vi "Datasheet Generate (Dynamic).vi"(4 "Generator Settings":T3, 8 "error in (no error)":errorcluster, 10 "Templates":string[](array[string]), 11 "Items":T2[](array[typedef])) -> (0 "error out":errorcluster, 2 "Actual (sec)":i32, 3 "Datasheet Paths":T1[](array[typedef]))   [LabVIEW 2011]
uses:
  Datasheet Generator Settings.ctl
  www/cgi-bin/_cgi-lib/TDM_INDEX Record.ctl
  Datasheet Report Info.ctl
  Datasheet Inputs.ctl
  Datasheet Outputs.ctl
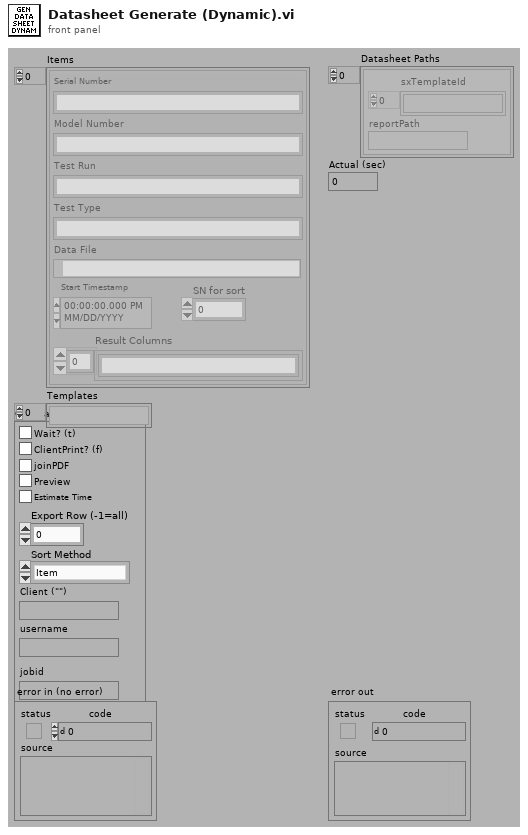
[diagram p1: front panel]
types:
  T1 = typedef "Datasheet Report Info.ctl" = cluster{"sxTemplateId":string[], "reportPath":path}
  T2 = typedef "TDM_INDEX Record.ctl" = cluster{"Model Number":string, "SN for sort":i32, "Test Type":string, "Test Run":string, "Serial Number":string, "Start Timestamp":timestamp, "Data File":path, "Result Columns":string[]}
  T3 = typedef "DATASHEET Generator Settings.ctl" = cluster{"Wait? (t)":bool, "ClientPrint? (f)":bool, "Client (\"\")":string, "joinPDF":bool, "Sort Method":enum16{"Item", "Template", "No Sort"}, "Export Row (-1=all)":i32, "Preview":bool, "Estimate Time":bool, "username":string, "jobid":string}
  T4 = typedef "Datasheet Outputs.ctl" = cluster{"Datasheet Paths":T5[], "Actual (Sec)":i32, "error out":errorcluster}
  T5 = typedef "DATASHEET Report Info.ctl" = cluster{"sxTemplateId":string[], "reportPath":path}
  T6 = typedef "DATASHEET INPUTS.ctl" = cluster{"Items":T2[], "Templates":string[], "Generator Settings":T3, "Response Queue Name":string}
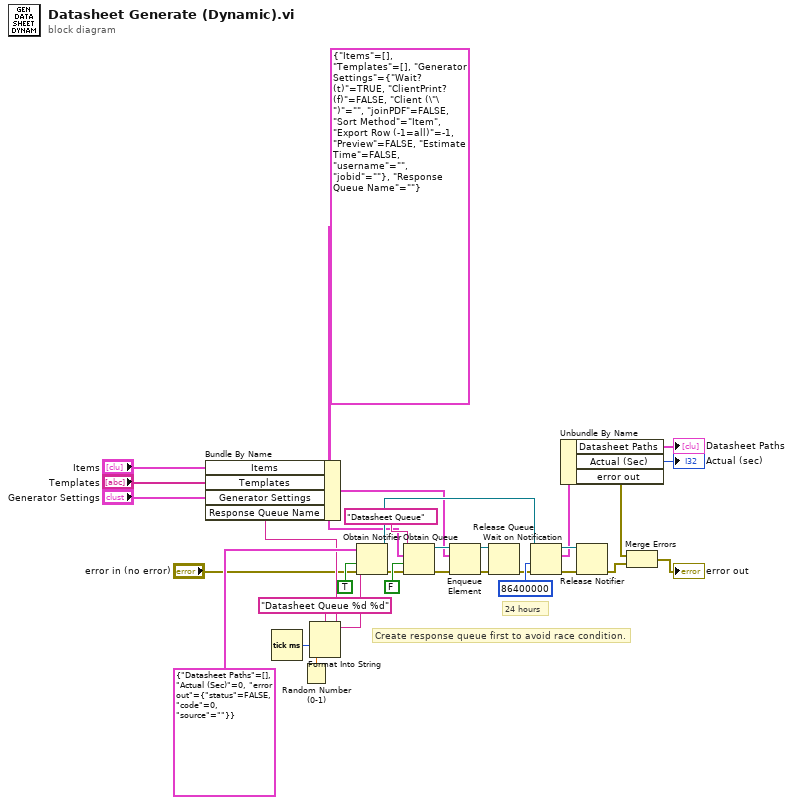
[diagram p0: block diagram]
diagram:
  w2 = T6 {"Items"=[], "Templates"=[], "Generator Settings"={"Wait? (t)"=TRUE, "ClientPrint? (f)"=FALSE, "Client (\"\")"="", "joinPDF"=FALSE, "Sort Method"=enum."Item", "Export Row (-1=all)"=-1, "Preview"=FALSE, "Estimate Time"=FALSE, "username"="", "jobid"=""}, "Response Queue Name"=""} ("INPUTS")
  # "Create response queue first to avoid race condition."
  # "24 hours"
  n1 = Tick Count (ms)() -> (millisecond timer value=w18:u32)
  n2 = Random Number (0-1)() -> (number: 0 to 1=w11:dbl)
  n3 = Format Into String(format string="Datasheet Queue %d %d" ("name (unnamed)"), w18, w11) -> (resulting string=w10:string)  [unwired: 2 in, 1 out]
  n4 = Bundle By Name(cluster=w2, "Items"="Items", "Templates"="Templates", "Generator Settings"="Generator Settings", "Response Queue Name"=w10) -> (w3:T6)
  n5 = Obtain Notifier(name (unnamed)=w10, notification data type=T4 {"Datasheet Paths"=[], "Actual (Sec)"=0, "error out"={"status"=FALSE, "code"=0, "source"=""}} ("OUTPUTS"), create if not found? (T)=TRUE, error in (no error)="error in (no error)") -> (notifier out=w29:refnum<notifier>, error out=w6:errorcluster)  [unwired: 1 out]
  n6 = Obtain Queue(name (unnamed)="Datasheet Queue", element data type=w2, create if not found? (T)=FALSE, error in (no error)=w6) -> (queue out=w23:refnum<queue>, error out=w24:errorcluster)  [unwired: 1 in, 1 out]
  n7 = Enqueue Element(queue=w23, element=w3, error in (no error)=w24) -> (queue out=w25:refnum<queue>, error out=w26:errorcluster)  [unwired: 1 in, 1 out]
  n8 = Release Queue(queue=w25, error in (no error)=w26) -> (error out=w1:errorcluster)  [unwired: 1 in, 2 out]
  n9 = Wait on Notification(notifier=w29, timeout in ms (-1)=86400000, error in (no error)=w1) -> (notifier out=w28:refnum<notifier>, notification=w17:T4, error out=w27:errorcluster)  [unwired: 1 in, 1 out]
  n10 = Unbundle By Name(w17) -> ("Datasheet Paths"=→"Datasheet Paths":T5[], "Actual (Sec)"=→"Actual (sec)":i32, "error out"=w8:errorcluster)
  n11 = Release Notifier(notifier=w28, error in (no error)=w27) -> (error out=w9:errorcluster)  [unwired: 1 in, 2 out]
  n12 = Merge Errors(w8, w9) -> (→"error out":errorcluster)
